vi "Table_LimitSettings.vi"(8 "error in":errorcluster, 11 "file path (use dialog)":path) -> (0 "error out":errorcluster, 3 "Limit Settings":variant)   [LabVIEW 2012, in "TableSupportLib.lvlib"]
uses:
  TableSupportLib.lvlib
  Table_LimitSettings.ctl
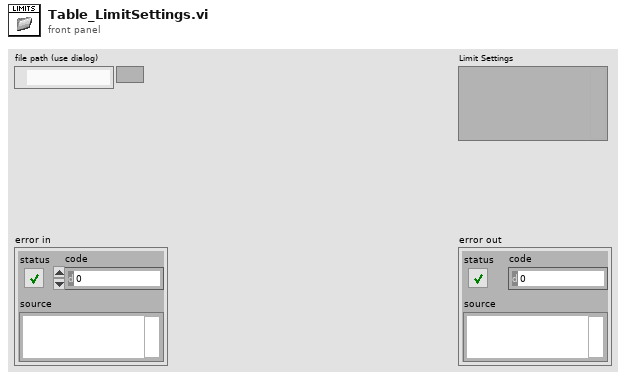
[diagram p1: front panel]
types:
  T1 = typedef "TableSupportLib.lvlib/Table_LimitSettings.ctl" = cluster{"High":dbl, "High Warning":dbl, "Low Warning":dbl, "Low":dbl}
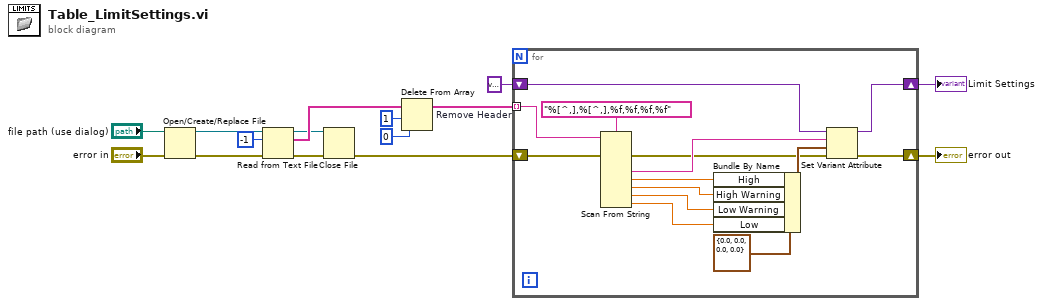
[diagram p0: block diagram]
diagram:
  n1 = Open/Create/Replace File(file path (use dialog)="file path (use dialog)", error in="error in") -> (refnum out=w13:refnum<file>, error out=w14:errorcluster)  [unwired: 4 in, 1 out]
  n2 = Read from Text File(file (use dialog)=w13, count=-1, error in=w14) -> (refnum out=w3:refnum<file>, text=w11:string[], error out=w2:errorcluster)  [unwired: 1 in, 1 out]
  n3 = Close File(refnum=w3, error in=w2) -> (error out=w1:errorcluster)  [unwired: 1 out]
  n4 = Delete From Array "Remove Header"(array=w11, length=1, index=0) -> (array with subset deleted=w8:string[])  [unwired: 1 out]
  n5 = for {
    tunnel: w8 -> [w28] mode=indexing
    shift-right: [w19] -> w6
    shift-left: variant ("variant") -> [w29]
    shift-right: [w17] -> w5
    shift-left: w1 -> [w16]
    n6 = Scan From String(format string="%[^,],%[^,],%f,%f,%f,%f", input string=w28, error in=w16) -> (error out=w18:errorcluster, output 2=w26:string, output 3=w24:dbl, output 4=w23:dbl, output 5=w22:dbl, output 6=w21:dbl)  [unwired: 8 in, 2 out]
    n7 = Bundle By Name(cluster=T1 {"High"=0.0, "High Warning"=0.0, "Low Warning"=0.0, "Low"=0.0}, "High"=w24, "High Warning"=w23, "Low Warning"=w22, "Low"=w21) -> (w20:T1)
    n8 = Set Variant Attribute(Variant=w29, name=w26, value=w20, error in=w18) -> (Variant out=w19:variant, error out=w17:errorcluster)  [unwired: 1 out]
  }
  "Limit Settings" <- w6
  "error out" <- w5
